vi "COMI SD502 Get Clk Freq.vi"(11 "nClkSrcIdx":i32) -> (3 "function return":dbl)   [LabVIEW 2017, in "Comidll.lvlib"]
doc: "double (COMI_SD502_GetClkFreq) (int nClkSrcIdx);"
uses:
  <userlib>/Comidll/Comidll.lvlib
  <userlib>/Comidll/Comidll.dll
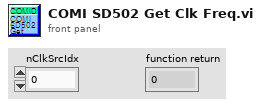
[diagram p1: front panel]
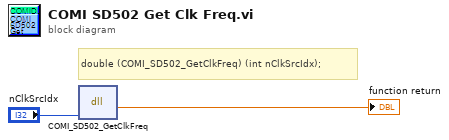
[diagram p0: block diagram]
diagram:
  # "double\t(COMI_SD502_GetClkFreq) (int nClkSrcIdx);"
  n1 = dll-call lib="C:/Program Files/National Instruments/LabVIEW 2017/user.lib/Comidll/Comidll.*" fn="COMI_SD502_GetClkFreq"("nClkSrcIdx"="nClkSrcIdx") -> (→"function return":dbl)  [unwired: 4 in, 2 out]
